vi "terminate.vi"(8 "error in (no error)":errorcluster, 11 "FPGA_AK101022Resonance in":refnum<class "FPGAWrapperAK101022Resonance.lvclass">) -> (0 "error out":errorcluster, 3 "FPGA_AK101022Resonance out":refnum<class "FPGAWrapperAK101022Resonance.lvclass">)   [LabVIEW 2010, in "FPGAWrapperAK101022Resonance.lvclass"]
uses:
  FPGAWrapperAK101022Resonance.lvclass
  GenericFPGAWrapper/GenericFPGAWrapper/GenericFPGAWrapper.lvclass
  class_data.vi
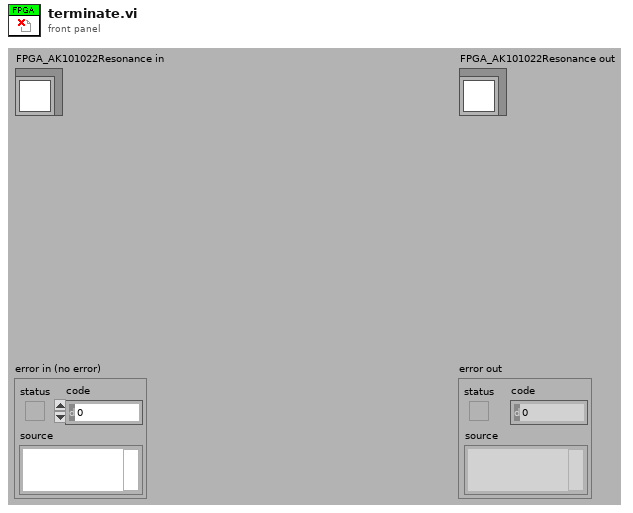
[diagram p1: front panel]
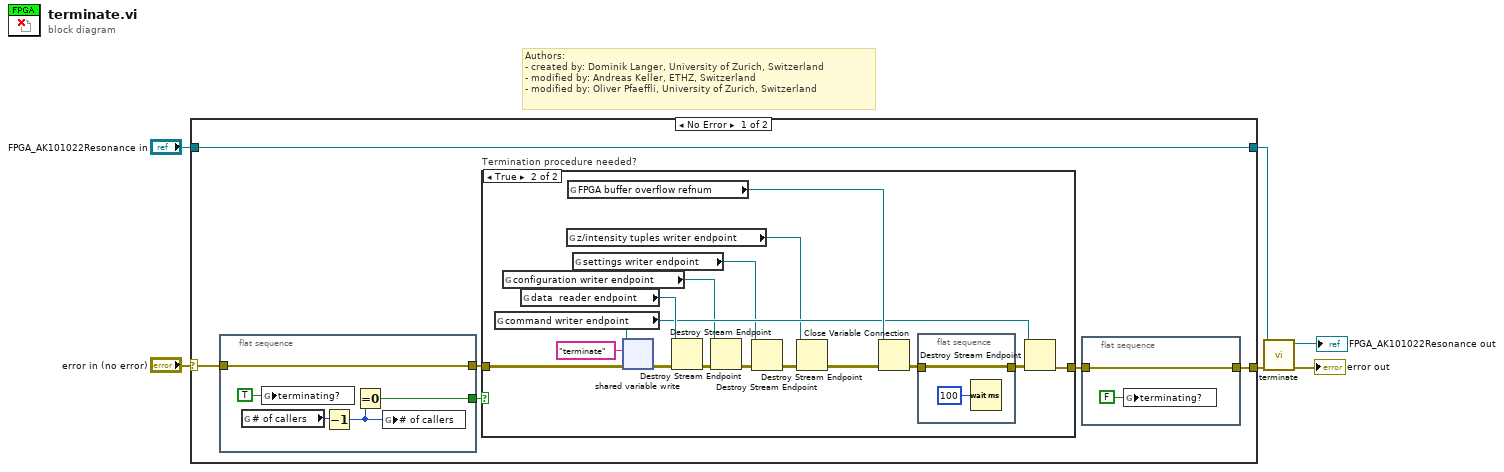
[diagram p0: block diagram]
diagram:
  # "Authors: \n- created by: Dominik Langer, University of Zurich, Switzerland\n- modified by: Andreas Keller, ETHZ, Switzerland\n- modified by: Oliver Pfaeffli, University of Zurich, Switzerland"
  n1 = case shown="No Error" "error in (no error)" {
    selector: "error in (no error)" -> [w11 w40]
    tunnel: "FPGA_AK101022Resonance in" -> [w12 w39]
    tunnel: [w7 w40] -> w3
    tunnel: [w12 w39] -> w1
    frame No Error {
      n2 = flat-sequence {
        tunnel: w11 -> [w17]
        tunnel: [w17] -> w10
        tunnel: [w15] -> w9
        frame #0 {
          n3 = global read "class_data.vi" "# of callers"() -> (w18:i32)
          n4 = global write "class_data.vi" "terminating?"(TRUE ("terminating?")) -> ()
          n5 = Decrement(x=w18) -> (x-1=w16:i32)
          n6 = Equal To 0?(x=w16) -> (x = 0?=w15:bool)
          n7 = global write "class_data.vi" "# of callers"(w16) -> ()
        }
      }
      n8 = case "Termination procedure needed?" shown="True" w9 {
        tunnel: [w20 w28] -> w8
        tunnel: w10 -> [w20 w35]
        frame False {
        }
        frame True {
          n9 = global read "class_data.vi" "command writer endpoint"() -> (w29:refnum<k21>)
          n10 = global read "class_data.vi" "configuration writer endpoint"() -> (w27:refnum<k21>)
          n11 = global read "class_data.vi" "data  reader endpoint"() -> (w36:refnum<k21>)
          n12 = global read "class_data.vi" "z/intensity tuples writer endpoint"() -> (w22:refnum<k21>)
          n13 = global read "class_data.vi" "FPGA buffer overflow refnum"() -> (w33:refnum<k21>)
          n14 = global read "class_data.vi" "settings writer endpoint"() -> (w24:refnum<k21>)
          n15 = shared-variable-write(w29, w35, "terminate" ("data in")) -> (w32:errorcluster)  [unwired: 1 in, 2 out]
          n16 = Destroy Stream Endpoint(8:w32, 11:w36) -> (0:w26:errorcluster)
          n17 = Destroy Stream Endpoint(8:w26, 11:w27) -> (0:w25:errorcluster)
          n18 = Destroy Stream Endpoint(8:w25, 11:w24) -> (0:w23:errorcluster)
          n19 = Destroy Stream Endpoint(8:w23, 11:w22) -> (0:w21:errorcluster)
          n20 = Close Variable Connection(8:w21, 11:w33) -> (0:w31:errorcluster)
          n21 = flat-sequence {
            tunnel: w31 -> [w37]
            tunnel: [w37] -> w30
            frame #0 {
              n22 = Wait (ms)(milliseconds to wait=u32 100) -> ()  [unwired: 1 out]
            }
          }
          n23 = Destroy Stream Endpoint(8:w30, 11:w29) -> (0:w28:errorcluster)
        }
      }
      n24 = flat-sequence {
        tunnel: w8 -> [w13]
        tunnel: [w13] -> w7
        frame #0 {
          n25 = global write "class_data.vi" "terminating?"(FALSE ("terminating?")) -> ()
        }
      }
    }
    frame Error {
    }
  }
  n26 = call-parent "terminate.vi"("error in (no error)"=w3, "GenericPlugin in"=w1) -> ("error out"=→"error out":errorcluster, "GenericPlugin out"=→"FPGA_AK101022Resonance out":refnum<class "FPGAWrapperAK101022Resonance.lvclass">)  [unwired: 8 in]
